vi "Get Connection Information Dialog.vi"(8 "error in (no error)":errorcluster, 9 "previous attempt error (no error)":errorcluster, 11 "Connection Info":T1={"VISA Resource"="", "Address"=1} {"Address" min=1}) -> (0 "error out":errorcluster, 2 "Cancelled?":bool, 3 "Connection Info out":T1={"VISA Resource"="", "Address"=1} {"Address" min=1})   [LabVIEW 2020, in "plugin_flodx_pressure.lvlib" / "plugin.lvlib"]
doc: "Asks the user for new connection information. The connection info is not validated here and needs to be sent back to the instrument validation to try the connection."
uses:
  plugin.lvlib
  Instrument Manager/connection_info/Connection Info.ctl
  Instrument Manager/Instrument Manager.lvlib
panel:
  in  "Address":i8=1
  in  "Cancel Btn":bool
  in  "VISA Resource/Comm Port":refnum<visa-resource-name>
  in  "Connect Btn":bool
  # "Set Connection Information"
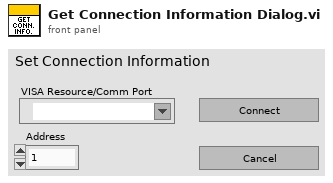
[diagram p1: front panel]
types:
  T1 = typedef "plugin_flodx_pressure.lvlib/plugin.lvlib/Instrument Manager.lvlib/Connection Info.ctl" = cluster{"VISA Resource":refnum<visa-resource-name>, "Address":u8}
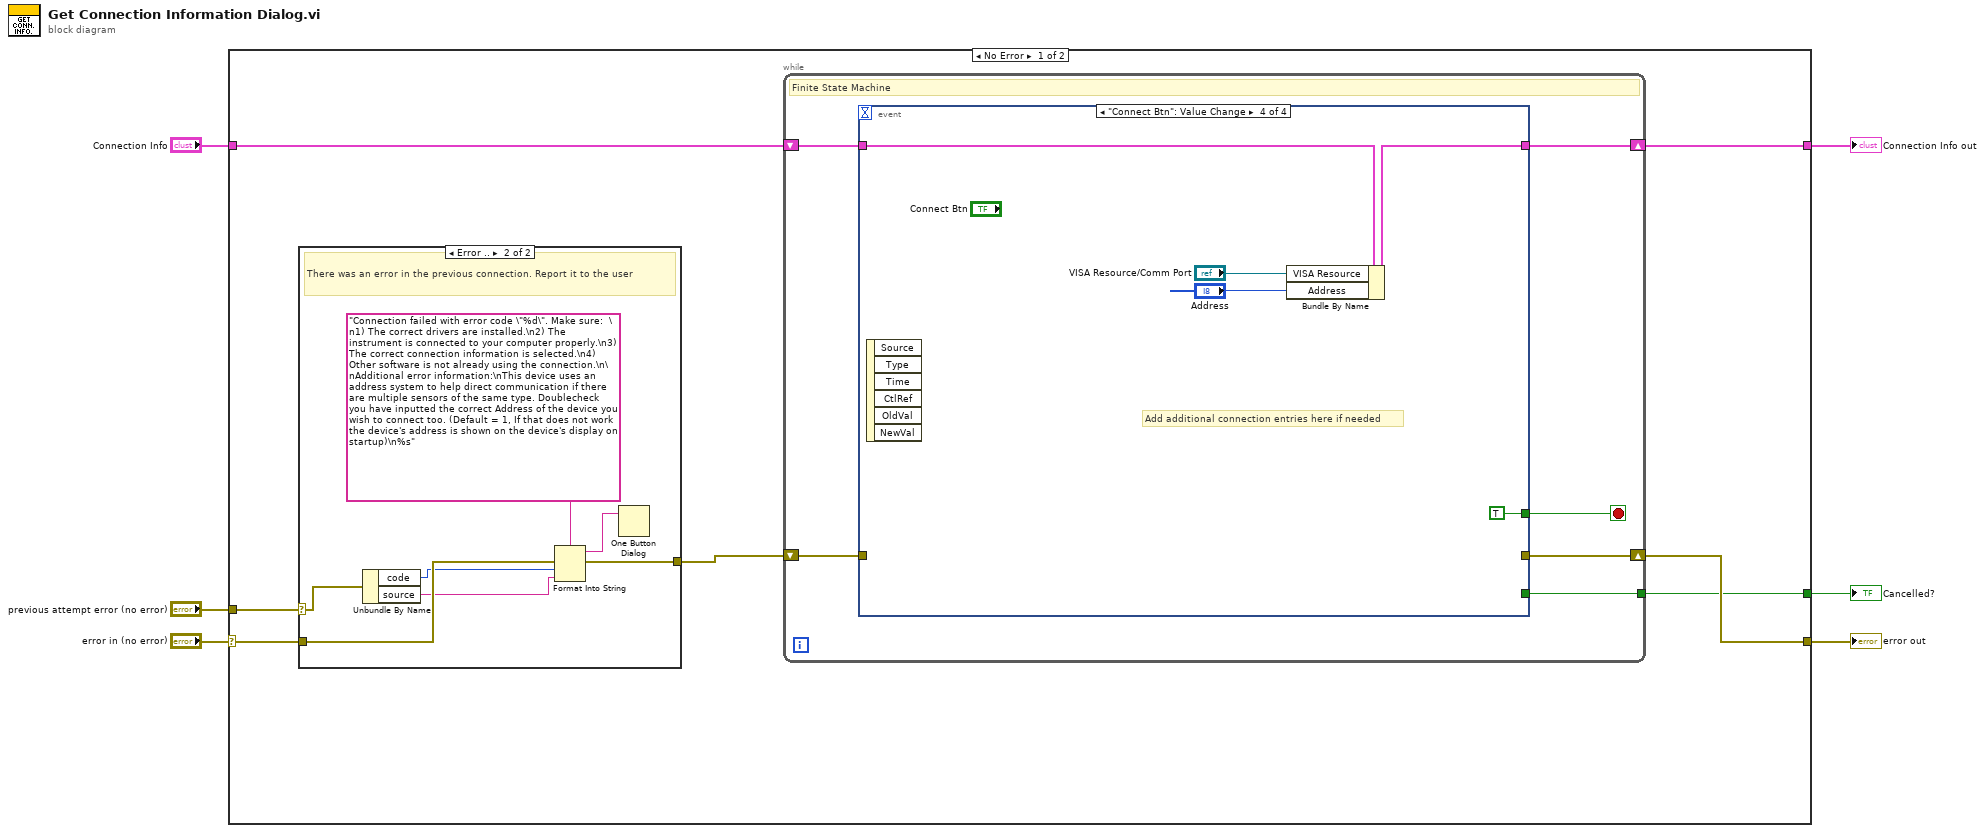
[diagram p0: block diagram]
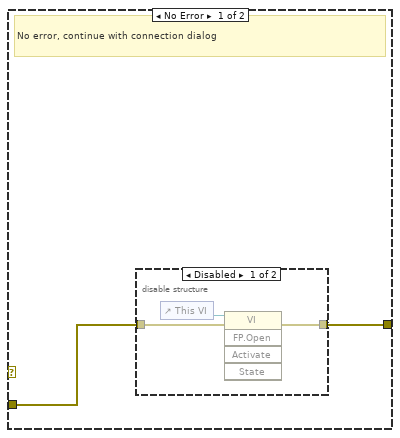
[diagram p2: hidden frame]
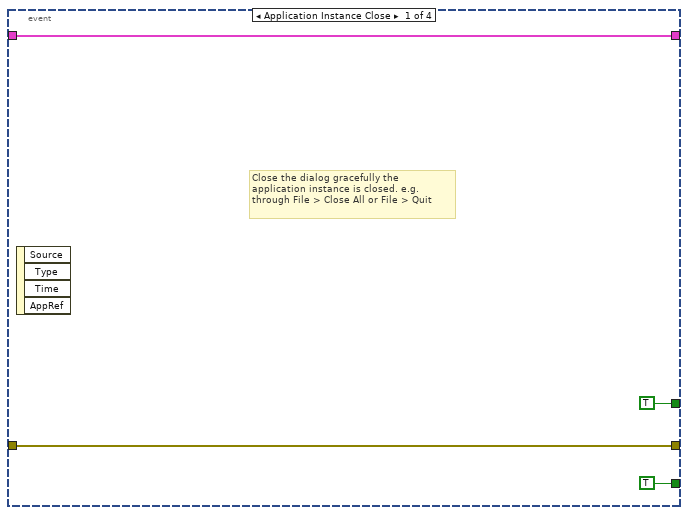
[diagram p4: hidden frame]
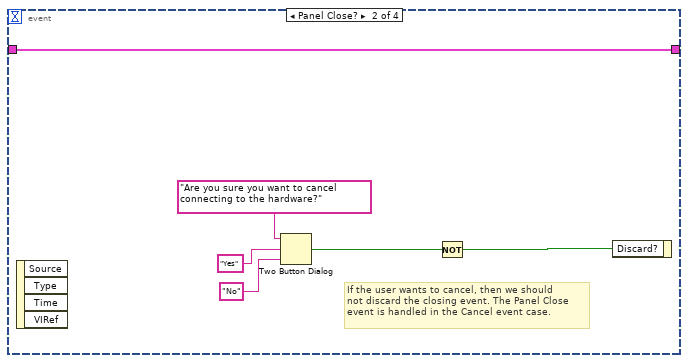
[diagram p5: hidden frame]
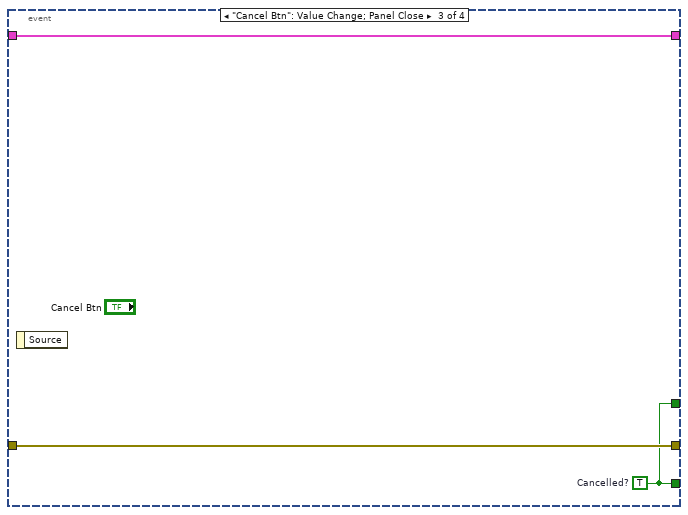
[diagram p6: hidden frame]
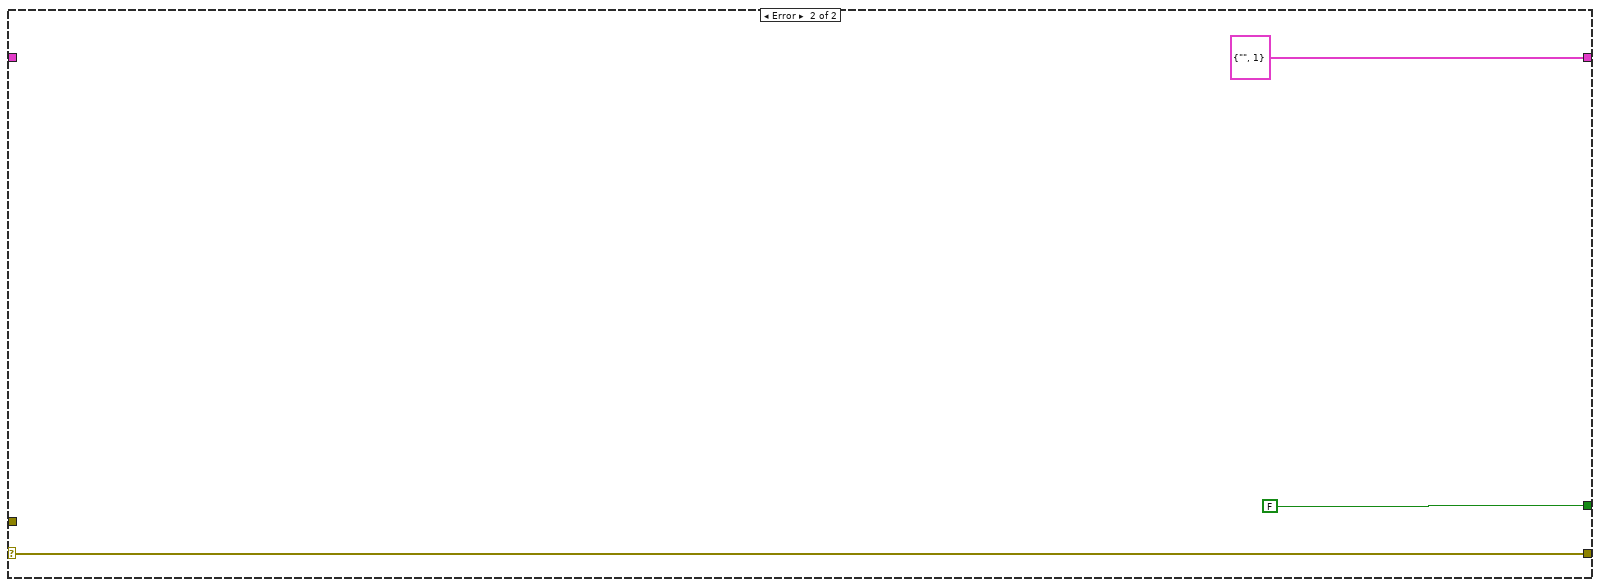
[diagram p7: hidden frame]
diagram:
  n1 = case shown="No Error" "error in (no error)" {
    selector: "error in (no error)" -> [w11 w53]
    tunnel: [w13 T1 {"VISA Resource"="", "Address"=1} ("Connection Info")] -> w3
    tunnel: [w12 w53] -> w5
    tunnel: "Connection Info" -> [w7 _]
    tunnel: [w9 FALSE ("Cancelled?")] -> w2
    tunnel: "previous attempt error (no error)" -> [w8 _]
    frame No Error {
      n2 = case shown="Error .." w8 {
        selector: w8 -> [_ w22]
        tunnel: w11 -> [w15 w23]
        tunnel: [w14 w24] -> w10
        frame No Error {
          # "No error, continue with connection dialog"
          n3 = disable-structure shown="Disabled" {
            disable-tunnel: w15 -> [w17 w19]
            disable-tunnel: [w16 w19] -> w14
            frame Disabled {
              n4 = control-ref of="This VI"() -> (w18:refnum<vi>)
              n5 = invoke class="VI" method="FP.Open"(reference=w18, error in=w17) -> (error out=w16:errorcluster)  [unwired: 3 in, 4 out]
            }
            frame Enabled {
            }
          }
        }
        frame Error {
          # "There was an error in the previous connection. Report it to the user"
          n6 = Unbundle By Name(w22) -> ("code"=w21:i32, "source"=w20:string)
          n7 = Format Into String(format string="Connection failed with error code \"%d\". Make sure:  \n1) The correct drivers are installed.\n2) The instrument is connected to your computer properly.\n3) The correct connection information is selected.\n4) Other software is not already using the connection.\n\nAdditional error information:\nThis device uses an address system to help direct communication if there are multiple sensors of the same type. Doublecheck you have inputted the correct Address of the device you wish to connect too. (Default = 1, If that does not work the device's address is shown on the device's display on startup)\n%s" ("message"), error in=w23, w21, w20) -> (resulting string=w25:string, error out=w24:errorcluster)  [unwired: 1 in]
          n8 = One Button Dialog(message=w25) -> ()  [unwired: 1 in, 1 out]
        }
      }
      n9 = while {
        shift-right: [w32] -> w13
        shift-left: w7 -> [w31]
        shift-right: [w28] -> w12
        shift-left: w10 -> [w29]
        tunnel: [w30] -> w9
        stop <- w27 stop-if-true
        # "Finite State Machine"
        n10 = event shown="[3] \"Connect Btn\": Value Change" {
          selector: _ -> [_ _ _ _]
          dyn-events: _ -> [_ _ _ _]
          timeout: _ -> [_ _ _ _]
          tunnel: [w36 w37 w45 w49] -> w32
          tunnel: w31 -> [w36 w37 w45 w50]
          tunnel: [TRUE ("Cancelled?") _ w43 _] -> w30
          tunnel: w29 -> [w35 _ w44 _]
          tunnel: [w35 _ w44 _] -> w28
          tunnel: [TRUE ("Cancelled?") _ w43 TRUE ("Cancelled?")] -> w27
          event Application Instance Close {
            # "Close the dialog gracefully the application instance is closed. e.g. through File > Close All or File > Quit"
            n11 = event-data() -> ()  [unwired: 1 in, 4 out]
          }
          event Panel Close? {
            # "If the user wants to cancel, then we should\nnot discard the closing event. The Panel Close\nevent is handled in the Cancel event case."
            n12 = event-data() -> ()  [unwired: 1 in, 4 out]
            n13 = Two Button Dialog(message="Are you sure you want to cancel connecting to the hardware?", 1:"No" ("F button name (\"Cancel\")"), 2:"Yes" ("T button name (\"OK\")")) -> (T button?=w40:bool)
            n14 = Not(x=w40) -> (.not. x?=w39:bool)
            n15 = event-data("Discard?"=w39) -> ()  [unwired: 1 in, 1 out]
          }
          event "Cancel Btn": Value Change; Panel Close {
            w43 = TRUE  # Cancelled?
            n16 = event-data() -> ()  [unwired: 1 in, 1 out]
          }
          event "Connect Btn": Value Change {
            # "Add additional connection entries here if needed"
            n17 = event-data() -> ()  [unwired: 1 in, 6 out]
            n18 = Bundle By Name(cluster=w50, "VISA Resource"="VISA Resource/Comm Port", "Address"="Address") -> (w49:T1)
          }
        }
      }
    }
    frame Error {
    }
  }
  "error out" <- w5
  "Connection Info out" <- w3
  "Cancelled?" <- w2
